vi "Horizontal Rod Sensor-State converter.vi"(0 "IN Sensor":bool, 2 "OUT Sensor":bool) -> (7 "Status":T1)   [LabVIEW 2016]
doc: "Takes IN/OUT sensor data and converts to state of horizontal rod:\n\nIN = TRUE; OUT = FALSE --> State = \"rod in\"\nIN = TRUE; OUT = TRUE --> State = \"status unclear\"\nIN = FALSE OUT = TRUE --> State = \"rod out\"\nIN = FALSE OUT = FALSE --> State = \"status unclear\""
uses:
  Horizontal Rod states.ctl
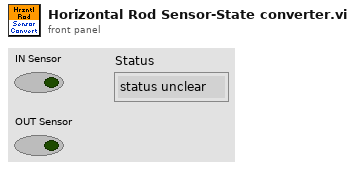
[diagram p1: front panel]
types:
  T1 = typedef "Horizontal Rod states.ctl" = enum16{"status unclear", "rod in", "rod out"}
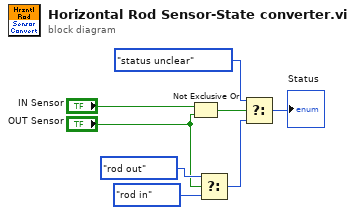
[diagram p0: block diagram]
diagram:
  n1 = Not Exclusive Or(1:"OUT Sensor", 2:"IN Sensor") -> (0:w1:bool)
  n2 = Select(t=Horizontal_Rod_states."rod out", s="OUT Sensor", f=Horizontal_Rod_states."rod in") -> (s? t:f=w6:T1)
  n3 = Select(t=Horizontal_Rod_states."status unclear", s=w1, f=w6) -> (s? t:f=→"Status":T1)
